vi "_SET_CONSTANTS.vi"() -> ()   [LabVIEW 2014]
uses:
  Events.vi
panel:
  in  "Exponential Drive Exponent":dbl=2.0
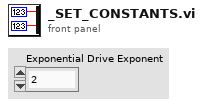
[diagram p1: front panel]
types:
  T1 = cluster{"Shooter latch power":dbl, "Shooter winch power":dbl, "Shooter gearbox servo angles disengaged":i32, "Shooter gearbox servo angles engaged":i32, "Shooter winch power while stalling":dbl, "Exponential Drive Exponent":dbl}
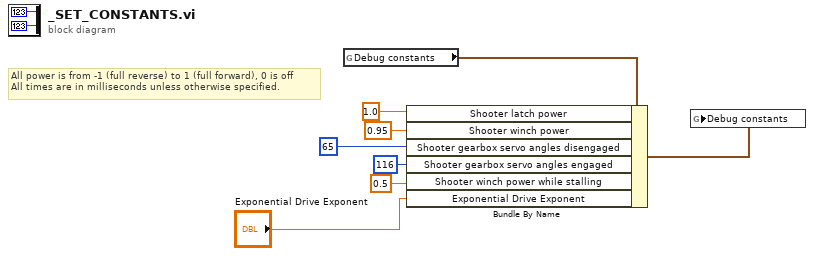
[diagram p0: block diagram]
diagram:
  # "All power is from -1 (full reverse) to 1 (full forward), 0 is off\nAll times are in milliseconds unless otherwise specified."
  n1 = global read "Events.vi" "Debug constants"() -> (w7:T1)
  n2 = Bundle By Name(cluster=w7, "Shooter latch power"=1.0, "Shooter winch power"=0.95, "Shooter gearbox servo angles disengaged"=65, "Shooter gearbox servo angles engaged"=116, "Shooter winch power while stalling"=0.5, "Exponential Drive Exponent"="Exponential Drive Exponent") -> (w8:T1)
  n3 = global write "Events.vi" "Debug constants"(w8) -> ()
